vi "TimerEngine.SetEngineStarted.vi"(8 "error in (no error)":errorcluster, 11 "data value reference":refnum<data-value>) -> (0 "error out":errorcluster, 3 "data value reference 2":refnum<data-value>)   [LabVIEW 2017, in "TimerEngine.lvlib" / "TimerEngine.lvclass"]
uses:
  TimerEngine.lvclass
  TimerEngine.lvclass/TimerEngine.ctl
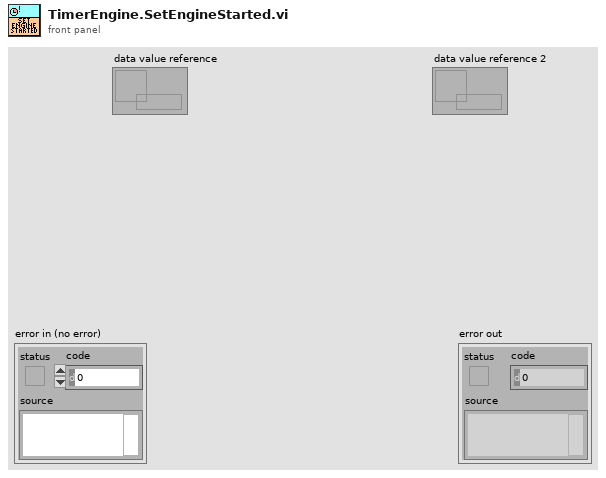
[diagram p1: front panel]
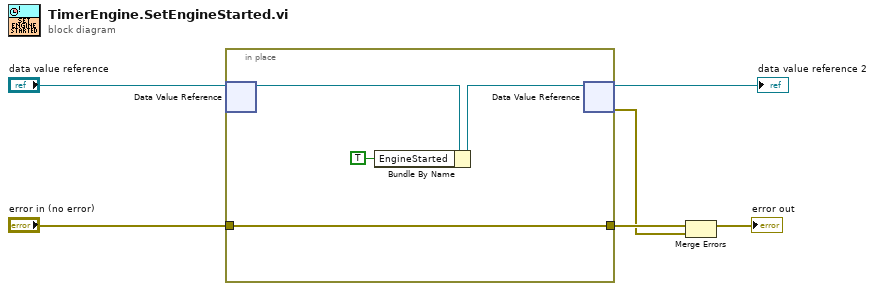
[diagram p0: block diagram]
diagram:
  n1 = in-place {
    in-place-border: [w9] -> w6
    in-place-border: "error in (no error)" -> [w9]
    n2 = in-place-dvr #1("data value reference") -> (w10:refnum<class "TimerEngine.lvclass">)  [unwired: 1 out]
    n3 = Bundle By Name(cluster=w10, "EngineStarted"=TRUE) -> (w8:refnum<class "TimerEngine.lvclass">)
    n4 = in-place-dvr #1(w8) -> (→"data value reference 2":refnum<data-value>, w3:errorcluster)
  }
  n5 = Merge Errors(w6, w3) -> (→"error out":errorcluster)
